vi "VG_MX5060.vi"() -> ()   [LabVIEW 2020]
panel:
  out "MX5060":string
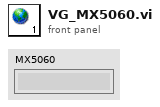
[diagram p1: front panel]
diagram:
